vi "CalculateZoomFactorAndOrigin__slk_mt.vi"(9 "bounds rectangle":T2, 11 "draw area size":cluster{"Width":u32, "Height":u32}) -> (1 "origin":T1, 3 "zoom factor":dbl)   [LabVIEW 2012, in "Lazyboots Menu Tool.lvlib" / "View__slk_mt.lvclass"]
doc: "Returns zoom factor an origin position."
uses:
  View__slk_mt.lvclass
  <vilib>/Utility/miscctls.llb/LVPointTypeDef.ctl
  <vilib>/Utility/miscctls.llb/LVRectTypeDef.ctl
panel:
  # "CalculateZoomFactorAndOrigin__slk_mt.vi\nReturns zoom factor an origin position.\n\nNOTICE -- YOU MUST LEAVE THIS NOTICE IN PLACE.\n\nCopyright (c) 2011, LIANG LIU Shawn.Liu.cn@gmail.com\nAll rights reserved.\n\nRedistribution and use in source and binary forms, with or without modification, are permitted provided that the following conditions are met:\n-Redistributions of source code must retain the above copyright notice, this list of conditions and the following disclaimer.\n-Redistributions in binary form must reproduce the above copyright notice, this list of conditions and the following disclaimer in the documentation and/or other materials provided with the distribution.\n-Neither the name of the eLp nor the names of its contributors may be used to endorse or promote products derived from this software without specific prior written permission.\n\nTHIS SOFTWARE IS PROVIDED BY THE COPYRIGHT HOLDERS AND CONTRIBUTORS \"AS IS\" AND ANY EXPRESS OR IMPLIED WARRANTIES, INCLUDING, BUT NOT LIMITED TO, THE IMPLIED WARRANTIES OF MERCHANTABILITY AND FITNESS FOR A PARTICULAR PURPOSE ARE DISCLAIMED. IN NO EVENT SHALL THE COPYRIGHT HOLDER OR CONTRIBUTORS BE LIABLE FOR ANY DIRECT, INDIRECT, INCIDENTAL, SPECIAL, EXEMPLARY, OR CONSEQUENTIAL DAMAGES (INCLUDING, BUT NOT LIMITED TO, PROCUREMENT OF SUBSTITUTE GOODS OR SERVICES; LOSS OF USE, DATA, OR PROFITS; OR BUSINESS INTERRUPTION) HOWEVER CAUSED AND ON ANY THEORY OF LIABILITY, WHETHER IN CONTRACT, STRICT LIABILITY, OR TORT (INCLUDING NEGLIGENCE OR OTHERWISE) ARISING IN ANY WAY OUT OF THE USE OF THIS SOFTWARE, EVEN IF ADVISED OF THE POSSIBILITY OF SUCH DAMAGE."
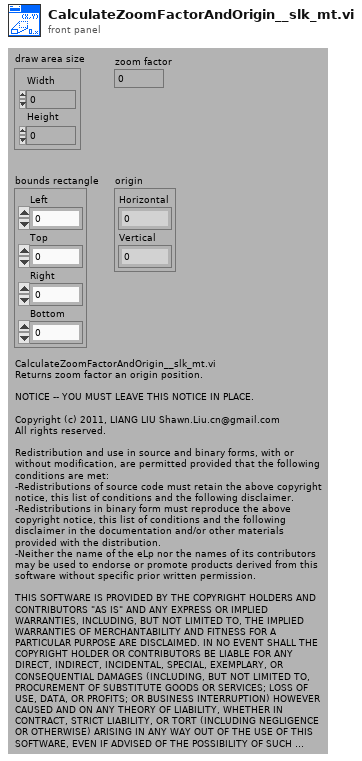
[diagram p1: front panel]
types:
  T1 = typedef "LVPointTypeDef.ctl" = cluster{"Horizontal":i16, "Vertical":i16}
  T2 = typedef "LVRectTypeDef.ctl" = cluster{"Left":i16, "Top":i16, "Right":i16, "Bottom":i16}
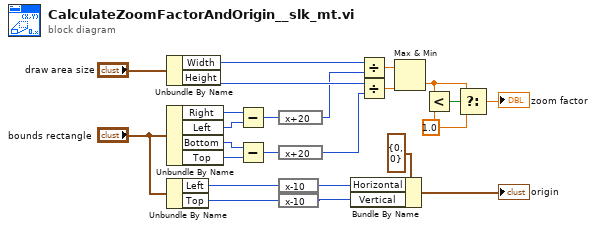
[diagram p0: block diagram]
diagram:
  w1 = 1.0 ("y")
  n1 = Unbundle By Name("draw area size") -> ("Width"=w15:u32, "Height"=w22:u32)
  n2 = Unbundle By Name("bounds rectangle") -> ("Right"=w18:i16, "Left"=w19:i16, "Bottom"=w21:i16, "Top"=w20:i16)
  n3 = Unbundle By Name("bounds rectangle") -> ("Left"=w12:i16, "Top"=w11:i16)
  n4 = Subtract(x=w18, y=w19) -> (x-y=w14:i16)
  n5 = Subtract(x=w21, y=w20) -> (x-y=w13:i16)
  n6 = expression code="x+20"(w14) -> (w6:i16)
  n7 = expression code="x+20"(w13) -> (w5:i16)
  n8 = expression code="x-10"(w12) -> (w8:i16)
  n9 = expression code="x-10"(w11) -> (w7:i16)
  n10 = Bundle By Name(cluster=T1 {"Horizontal"=0, "Vertical"=0} ("Origin"), "Horizontal"=w8, "Vertical"=w7) -> (→"origin":T1)
  n11 = Divide(x=w15, y=w6) -> (x/y=w23:dbl)
  n12 = Divide(x=w22, y=w5) -> (x/y=w24:dbl)
  n13 = Max & Min(x=w23, y=w24) -> (min(x,y)=w2:dbl)  [unwired: 1 out]
  n14 = Less?(x=w2, y=w1) -> (x < y?=w4:bool)
  n15 = Select(t=w2, s=w4, f=w1) -> (s? t:f=→"zoom factor":dbl)
